vi "Make Zernike Array v1.vi"(1 "size":u16, 2 "z":u8=9) -> (0 "zernike array":dbl[][](graph) caption="wrapped\ntheta")   [LabVIEW 2018]
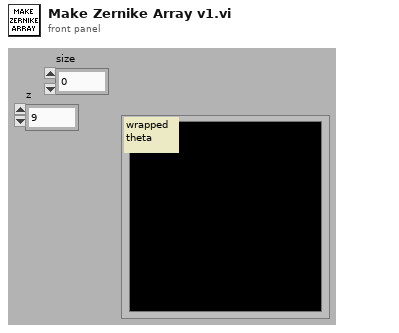
[diagram p1: front panel]
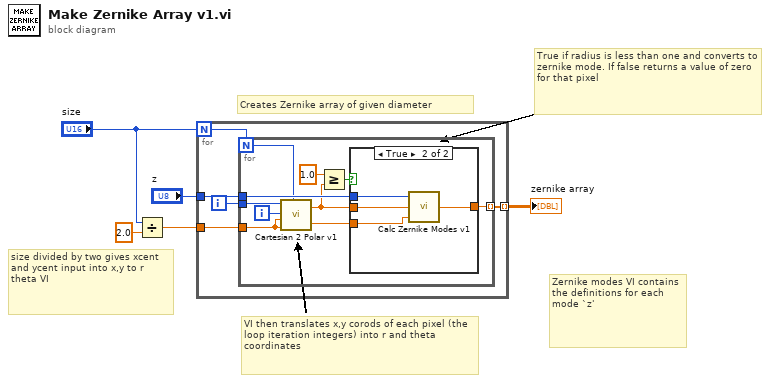
[diagram p0: block diagram]
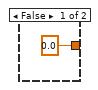
[diagram p2: hidden frame]
diagram:
  # "Zernike modes VI contains the definitions for each mode `z'"
  # "True if radius is less than one and converts to zernike mode. If false returns a value of zero for that pixel"
  # "VI then translates x,y corods of each pixel (the loop iteration integers) into r and theta coordinates"
  # "size divided by two gives xcent and ycent input into x,y to r theta VI"
  # "Creates Zernike array of given diameter"
  n1 = Divide(x="size", y=2.0) -> (x/y=w3:dbl)
  n2 = for {
    N: "size" -> [w6]
    tunnel: [w8] -> w2 mode=indexing
    tunnel: "z" -> [w9]
    tunnel: w3 -> [w7]
    i -> [w10]
    n3 = for {
      N: w6 -> [w11]
      tunnel: w10 -> [w19]
      tunnel: w9 -> [w17]
      tunnel: [w13] -> w8 mode=indexing
      tunnel: w7 -> [w12]
      i -> [w20]
      n4 = call "Cartesian 2 Polar v1.vi"("x"=w19, "y"=w20, "xcent"=w12, "ycent"=w12, "diam"=w11) -> ("rho"=w15:dbl, "theta"=w18:dbl)
      n5 = Greater Or Equal?(x=1.0, y=w15) -> (x >= y?=w16:bool)
      n6 = case shown="True" w16 {
        tunnel: w18 -> [_ w25]
        tunnel: w15 -> [_ w24]
        tunnel: w17 -> [_ w23]
        tunnel: [0.0 ("zernike") w22] -> w13
        frame False {
        }
        frame True {
          n7 = call "Calc Zernike Modes v1.vi"("t"=w25, "r"=w24, "z"=w23) -> ("zernike"=w22:dbl)
        }
      }
    }
  }
  "zernike array" <- w2
